vi "DHE.bak.vi"(0 "modpath":path, 7 "Cmd":string, 11 "error in":errorcluster) -> (4 "ImmedReplyString":string, 6 "DHE_DBSRef":T1, 10 "TimeOut out":i32, 15 "error out":errorcluster)   [LabVIEW 2016]
uses:
  DBSHAND/private/vis/DatabaseHand_RefNum.ctl
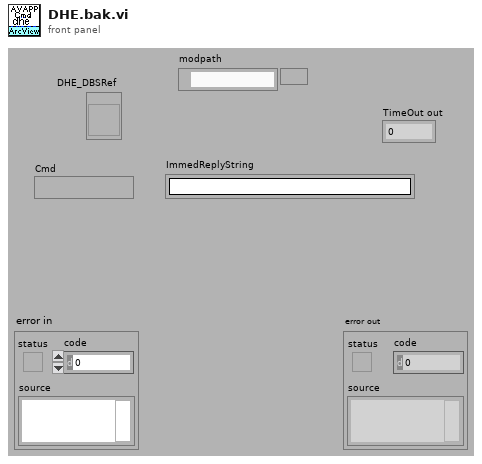
[diagram p1: front panel]
types:
  T1 = typedef "DatabaseHand_RefNum.ctl" = refnum<vi>
  T2 = typedef "DHE_Device.ctl" = cluster{"DevNo":i32, "fd":i32, "name":string, "FPA":string, "modifiers":string, "binpatt":string, "readtime":dbl, "readmode":string, "type":string, "params":string}
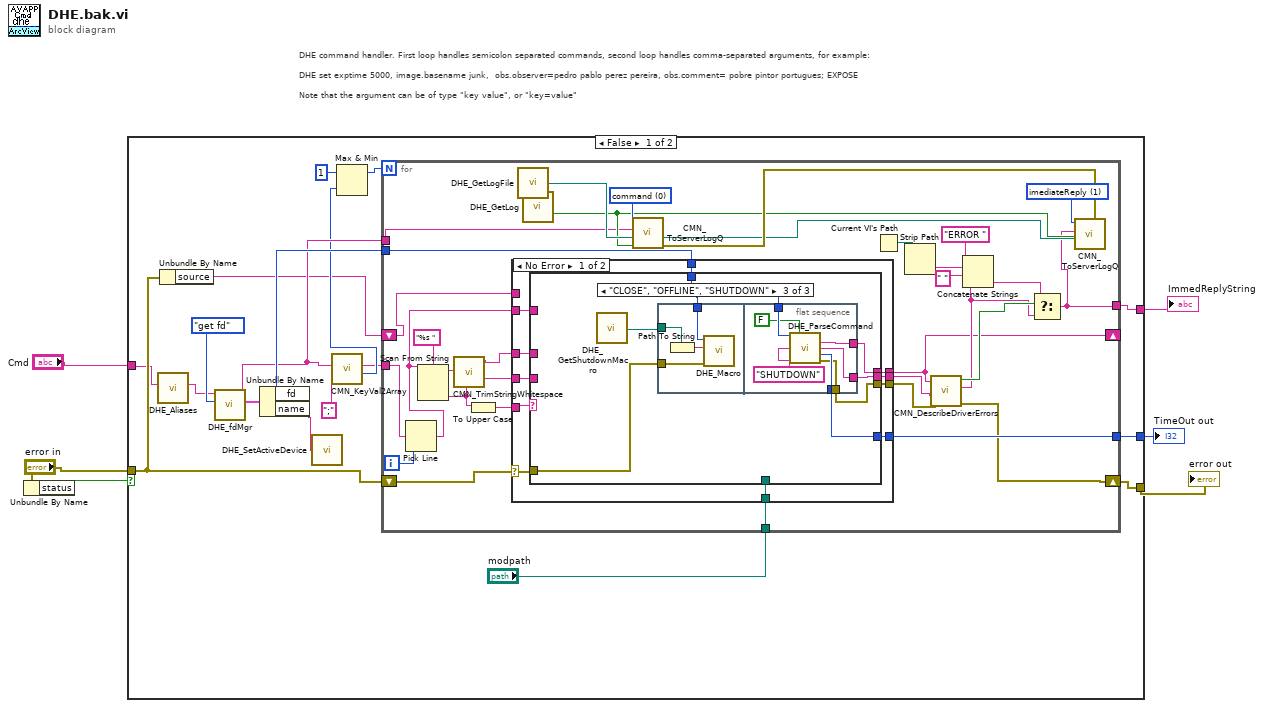
[diagram p0: block diagram]
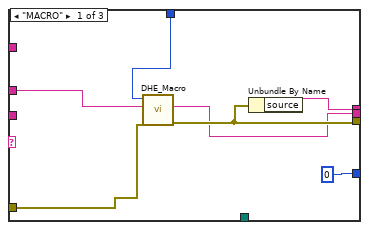
[diagram p2: hidden frame]
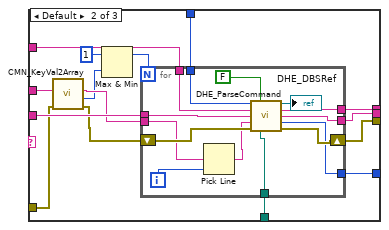
[diagram p3: hidden frame]
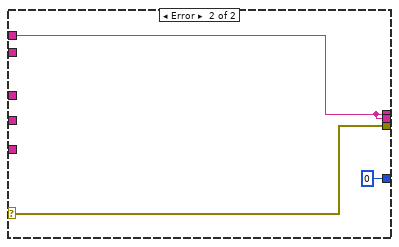
[diagram p4: hidden frame]
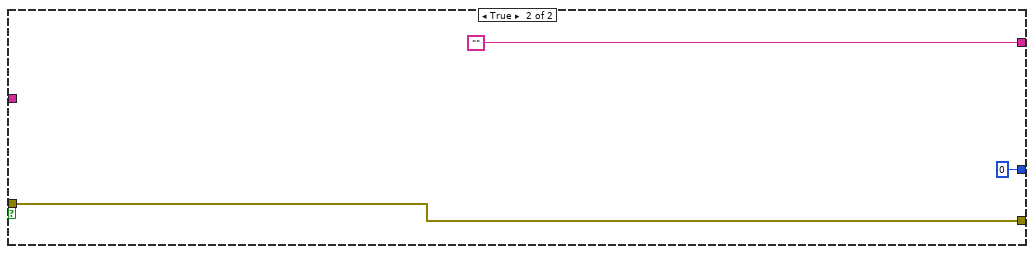
[diagram p5: hidden frame]
diagram:
  # "DHE command handler. First loop handles semicolon separated commands, second loop handles comma-separated arguments, for example:\n\nDHE set exptime 5000, image.basename junk,  obs.observer=pedro pablo perez pereira, obs.comment= pobre pintor portugues; EXPOSE\n\nNote that the argument can be of type \"key value\", or \"key=value\""
  n1 = Unbundle By Name("error in") -> ("status"=w3:bool)
  n2 = case shown="False" w3 {
    tunnel: "error in" -> [w11 w126]
    tunnel: [w14 w126] -> w6
    tunnel: [w12 ""] -> w5
    tunnel: "Cmd" -> [w8 _]
    tunnel: [w20 0 ("TimeOut out")] -> w1
    frame False {
      n3 = call "DHE_Aliases.vi"("name in"=w8) -> ("name out"=w7:string)  [unwired: 7 in, 3 out]
      n4 = Unbundle By Name(w11) -> ("source"=w10:string)
      n5 = call "DHE_fdMgr.vi"("action"=enum16{"get fd", "set fd"}."get fd", "cmd in"=w7) -> ("Device"=w23:T2, "cmd out"=w19:string)  [unwired: 3 in, 5 out]
      n6 = Unbundle By Name(w23) -> ("fd"=w22:i32, "name"=w21:string)
      n7 = call "DHE_SetActiveDevice.vi"("DHE_ActiveDevice"=w21) -> ()  [unwired: 9 out]
      n8 = call "CMN_KeyVal2Array.vi"("separator"=";", "command in"=w19) -> ("number of commands"=w18:i32, "commands out"=w13:string)  [unwired: 1 in, 6 out]
      n9 = Max & Min(x=1, y=w18) -> (max(x,y)=w15:i32)  [unwired: 1 out]
      n10 = for {
        N: w15 -> [_]
        tunnel: w22 -> [w43]
        tunnel: [w40] -> w20
        tunnel: w19 -> [w39]
        shift-right: [w33] -> w14
        shift-left: w11 -> [w29]
        tunnel: w13 -> [w32]
        tunnel: [w28] -> w12
        shift-right: [w27] -> _
        shift-left: w10 -> [w26]
        tunnel: "modpath" -> [w25]
        i -> [w31]
        w45 = u16 1 items=["command", "imediateReply", "Callback Reply", "Information"] ("type")
        w46 = u16 0 items=["command", "imediateReply", "Callback Reply", "Information"] ("type")
        n11 = Pick Line(multi-line string=w32, line index=w31) -> (output string=w30:string)  [unwired: 1 out]
        n12 = Scan From String(format string="%s " ("Format String"), input string=w30) -> (remaining string=w37:string, output 1=w36:string)  [unwired: 2 in, 3 out]
        n13 = call "CMN_TrimStringWhitespace.vi"("string"=w37) -> ("trimmed string"=w34:string)  [unwired: 1 in, 8 out]
        n14 = To Upper Case(1:w36) -> (0:w35:string)
        n15 = case shown="No Error" w29 {
          selector: w29 -> [w57 w123]
          tunnel: [w66 w121] -> w27
          tunnel: [w65 w123] -> w48
          tunnel: [w64 w121] -> w47
          tunnel: w43 -> [w63 _]
          tunnel: [w62 0 ("TimeOut out")] -> w40
          tunnel: w36 -> [w61 _]
          tunnel: w35 -> [w60 _]
          tunnel: w34 -> [w59 _]
          tunnel: w30 -> [w58 _]
          tunnel: w26 -> [_ w121]
          tunnel: w25 -> [w56 _]
          frame No Error {
            n16 = case shown="\"CLOSE\", \"OFFLINE\", \"SHUTDOWN\"" w60 {
              tunnel: w58 -> [_ w88 _]
              tunnel: w61 -> [_ w87 _]
              tunnel: [w71 w86 w106] -> w66
              tunnel: w59 -> [w69 w85 _]
              tunnel: w57 -> [w73 w84 w109]
              tunnel: [w72 w81 w103] -> w65
              tunnel: [w68 w78 w104] -> w64
              tunnel: w63 -> [w70 w76 w107]
              tunnel: [0 ("TimeOut out") w75 w105] -> w62
              tunnel: w56 -> [_ w74 _]
              frame "MACRO" {
                n17 = call "DHE_Macro.vi"("error in (no error)"=w73, "macro"=w69, "fd"=w70) -> ("error out"=w72:errorcluster, "response"=w68:string)  [unwired: 1 in, 6 out]
                n18 = Unbundle By Name(w72) -> ("source"=w71:string)
              }
              frame Default {
                n19 = call "CMN_KeyVal2Array.vi"("error in (no error)"=w84, "command in"=w85) -> ("error out"=w82:errorcluster, "number of commands"=w80:i32, "commands out"=w83:string)  [unwired: 1 in, 5 out]
                n20 = Max & Min(x=1, y=w80) -> (max(x,y)=w77:i32)  [unwired: 1 out]
                n21 = for {
                  N: w77 -> [_]
                  tunnel: w76 -> [w102]
                  tunnel: w88 -> [w101]
                  tunnel: w87 -> [w100]
                  tunnel: [w99] -> w86
                  tunnel: w83 -> [w95]
                  shift-right: [w97] -> w81
                  shift-left: w82 -> [w98]
                  tunnel: [w93] -> w78
                  tunnel: [w92] -> w75
                  tunnel: w74 -> [w90]
                  i -> [w96]
                  n22 = Pick Line(multi-line string=w95, line index=w96) -> (output string=w94:string)  [unwired: 1 out]
                  n23 = call "DHE_ParseCommand.vi"("fd"=w102, "Log"=FALSE, "command + args"=w101, "command"=w100, "arguments"=w94, "error in"=w98, "modpath"=w90) -> ("DHE_DBSRef"=→"DHE_DBSRef":T1, "message"=w99:string, "OK message"=w93:string, "TimeOut out"=w92:i32, "error out"=w97:errorcluster)  [unwired: 4 out]
                }
              }
              frame "CLOSE", "OFFLINE", "SHUTDOWN" {
                n24 = call "DHE_GetShutdownMacro.vi"() -> ("DHE_InitMacro"=w108:path)  [unwired: 9 out]
                n25 = flat-sequence {
                  tunnel: w109 -> [w113]
                  tunnel: w107 -> [w112]
                  tunnel: w108 -> [w111]
                  tunnel: w107 -> [w120]
                  tunnel: [w118] -> w106
                  tunnel: [w117] -> w105
                  tunnel: [w116] -> w104
                  tunnel: [w115] -> w103
                  frame #0 {
                    n26 = Path To String(path=w111) -> (string=w110:string)
                    n27 = call "DHE_Macro.vi"("error in (no error)"=w113, "macro"=w110, "fd"=w112) -> ()  [unwired: 1 in, 8 out]
                  }
                  frame #1 {
                    n28 = call "DHE_ParseCommand.vi"("fd"=w120, "Log"=FALSE, "command"="SHUTDOWN") -> ("message"=w118:string, "OK message"=w116:string, "TimeOut out"=w117:i32, "error out"=w115:errorcluster)  [unwired: 4 in, 5 out]
                  }
                }
              }
            }
          }
          frame Error {
          }
        }
        n29 = call "DHE_GetLogFile.vi"() -> ("DHE_LogFile"=w42:path)  [unwired: 9 out]
        n30 = call "DHE_GetLog.vi"() -> ("DHE_log"=w41:bool)  [unwired: 9 out]
        n31 = call "CMN_ToServerLogQ.vi"("Log"=w41, "file"=w42, "string"=w39, "type"=w46) -> ("error out"=w44:errorcluster)  [unwired: 2 in, 4 out]
        n32 = Current VI's Path() -> (path=w53:path)
        n33 = Strip Path(path=w53) -> (name=w52:string)  [unwired: 1 out]
        n34 = call "CMN_DescribeDriverErrors.vi"("message"=w27, "OK message"=w47, "error in (no error)"=w48) -> ("error?"=w50:bool, "astroerrors"=w49:string, "error out"=w33:errorcluster)  [unwired: 1 in, 4 out]
        n35 = Concatenate Strings("ERROR ", w52, " ", w49) -> (w54:string)
        n36 = Select(t=w54, s=w50, f=w49) -> (s? t:f=w28:string)
        n37 = call "CMN_ToServerLogQ.vi"("error in (no error)"=w44, "Log"=w41, "file"=w42, "string"=w28, "type"=w45) -> ()  [unwired: 1 in, 5 out]
      }
    }
    frame True {
    }
  }
  "error out" <- w6
  "ImmedReplyString" <- w5
  "TimeOut out" <- w1
